vi "Read Saftey Disable.vi"(0 "FPGA VI Reference in":T1, 3 "error in (no error)":errorcluster) -> (7 "FPGA VI Reference out":T1, 8 "GO":bool, 10 "error out":errorcluster)   [LabVIEW 2009]
uses:
  TypeDefs/Sensor TypeDefs/FPGA Main ref.ctl
  <vilib>/rvi/interface/nirviReadWriteControl/nirviReadWriteControl.xnode
  FPGA Bitfiles/Q_IGVC_2010.lvproj_FPGA Target_FPGA_MAIN.vi.lvbitx
  <vilib>/Utility/error.llb/Error Cluster From Error Code.vi
  <vilib>/rvi/errors/niLvFpgaAdjustHostInterfaceError.vi
  <vilib>/rvi/interface/common/niFpgaNodeNameForErrorReporting.ctl
  <vilib>/rvi/errors/niLvFpgaWhatHappensToTopLevelVI.ctl
  NiRioSrv.dll
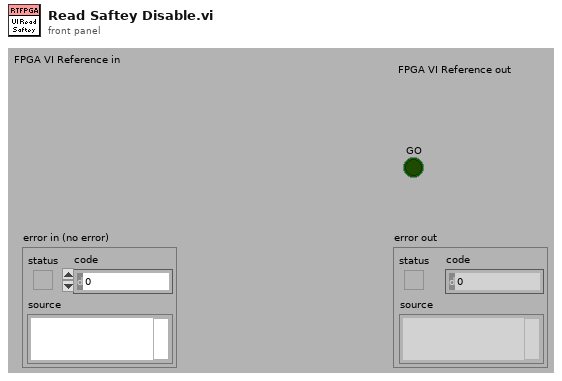
[diagram p1: front panel]
types:
  T1 = typedef "FPGA Main ref.ctl" = refnum<k20>
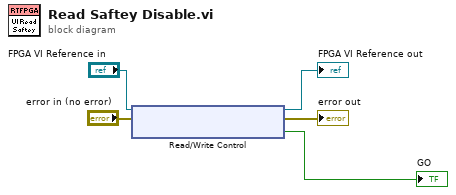
[diagram p0: block diagram]
diagram:
  n1 = xnode "Read/Write Control"("FPGA VI Reference In"="FPGA VI Reference in", "error in"="error in (no error)") -> ("FPGA VI Reference Out"=→"FPGA VI Reference out":T1, "error out"=→"error out":errorcluster, "Debounced Safety Switch"=→"GO":bool)
